vi "Destroy.vi"(8 "error in (no error)":errorcluster, 11 "reference in":refnum<class "SubTemplate_4x4x4.lvclass">) -> (0 "error out":errorcluster, 3 "reference out":refnum<class "SubTemplate_4x4x4.lvclass">)   [LabVIEW 2020, in "SubTemplate_4x4x4.lvclass"]
uses:
  <resource>/Framework/Providers/Open_GDS/ClassProviders/Provider_EndevoGOOP300/Templates/SubTemplate_4x4x4/SubTemplate_4x4x4.lvclass
  <resource>/Framework/Providers/Open_GDS/ClassProviders/Provider_EndevoGOOP300/Templates/BaseTemplate_4x4x4/BaseTemplate_4x4x4.lvclass
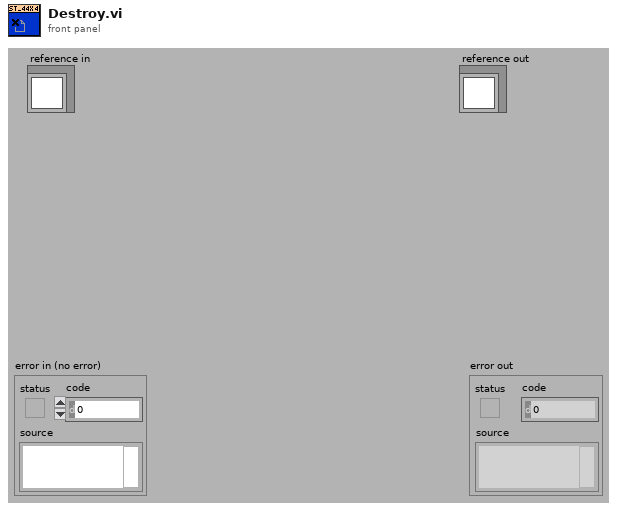
[diagram p1: front panel]
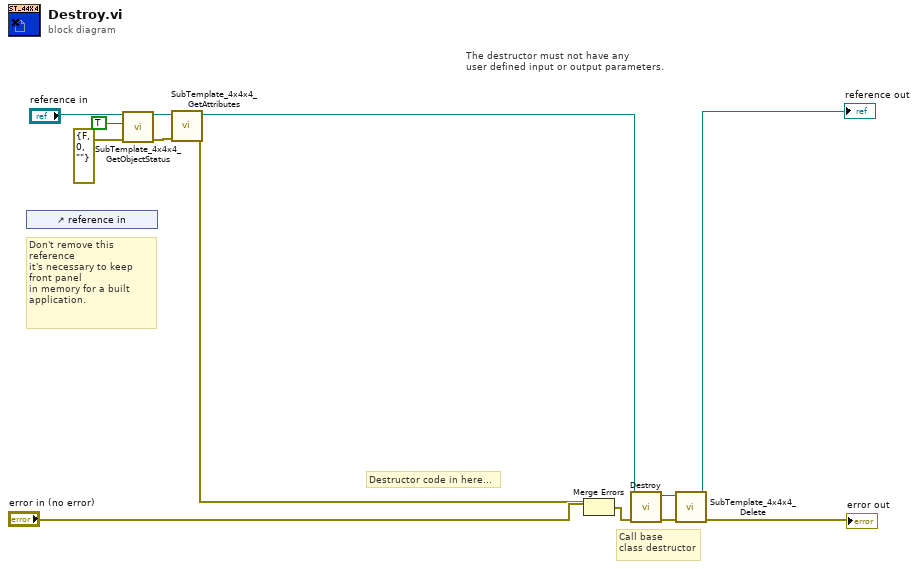
[diagram p0: block diagram]
diagram:
  # "Don't remove this reference\nit's necessary to keep front panel\nin memory for a built application."
  # "Destructor code in here..."
  # "The destructor must not have any\nuser defined input or output parameters."
  # "Call base\nclass destructor"
  n1 = control-ref of="reference in"() -> ()  [unwired: 1 out]
  n2 = call <resource>:"SubTemplate_4x4x4_GetObjectStatus.vi"("reference in"="reference in", "Simple Info"=TRUE, "error in (no error)"=errorcluster {"status"=FALSE, "code"=0, "source"=""}) -> ("reference out"=w9:refnum<class "SubTemplate_4x4x4.lvclass">, "error out"=w7:errorcluster)  [unwired: 3 in, 8 out]
  n3 = call <resource>:"SubTemplate_4x4x4_GetAttributes.vi"("error in (no error)"=w7, "reference in"=w9) -> ("error out"=w10:errorcluster, "reference out"=w3:refnum<class "SubTemplate_4x4x4.lvclass">)  [unwired: 6 in, 2 out]
  n4 = Merge Errors("error in (no error)", w10) -> (w4:errorcluster)
  n5 = call-parent "Destroy.vi"("error in (no error)"=w4, "reference in"=w3) -> ("error out"=w5:errorcluster, "reference out"=w2:refnum<class "SubTemplate_4x4x4.lvclass">)  [unwired: 8 in]
  n6 = call <resource>:"SubTemplate_4x4x4_Delete.vi"("error in (no error)"=w5, "reference in"=w2) -> ("error out"=→"error out":errorcluster, "reference out"=→"reference out":refnum<class "SubTemplate_4x4x4.lvclass">)  [unwired: 7 in, 1 out]
